vi "Customize VI Window.vi"() -> ()   [LabVIEW 2010]
doc: "This VI demonstrates VI Server methods and properties: Show Menu Bar, Show Title Bar, VI Transparency, and Centering the VI."
panel:
  in  "Center":bool
  in  "stop":bool
  in  "Make VI Transparent?":bool
  in  "Show Title Bar?":bool
  in  "Show Menu Bar?":bool
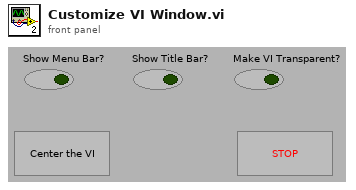
[diagram p1: front panel]
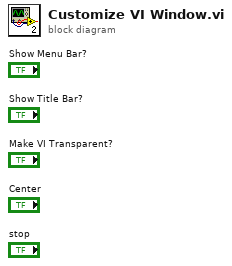
[diagram p0: block diagram]
diagram:
